vi "BSCAN_DEMO08_Zynq_W25Q128JV_registerRead_DeviceID_90h.vi"(8 "error in":errorcluster) -> (0 "error out":errorcluster, 4 "Data out":u8[](array[numeric]) format="%08b")   [LabVIEW 2017]
uses:
  Saldigi_protocol_library.lvlibp/SPI1_bitstream/SPI1_typedef.ctl
  Saldigi_protocol_library.lvlibp/HAL/HAL_version_typedef.ctl
  Saldigi_protocol_library.lvlibp
panel:
  in  "SPI1 typedef in":T1={"MOSI padded"=[], "CLK padded"=[], "-CS padded"=[], "String array"=[], "clocked bits"=0, "output rate"=0.0, "MOSI IO0 channel name"="chain0/xc7z020_clg400/PS_MIO2", "CLK channel name"="chain0/xc7z020_clg400/PS_MIO6", "MISO IO1 channel name"="chain0/xc7z020_clg400/PS_MIO3", "Parameter string"="", "-CS channel name"="chain0/xc7z020_clg400/PS_MIO1", "SPI mode"=enum."MODE 0", "Version"=enum."BSCAN V2"}
  in  "milliseconds to wait\nbetween iterations":u32
  out "dt":dbl(graph)=0.7297572000024957
  in  "stop":bool
  out "(ID7 - ID0) 17h":u8=23 format="%08b"
  out "(MF7 - MF0) EFh":u8=239 format="%08b"
  # "expected register values\nfrom datasheet"
  # "saldigi.fi protocol library"
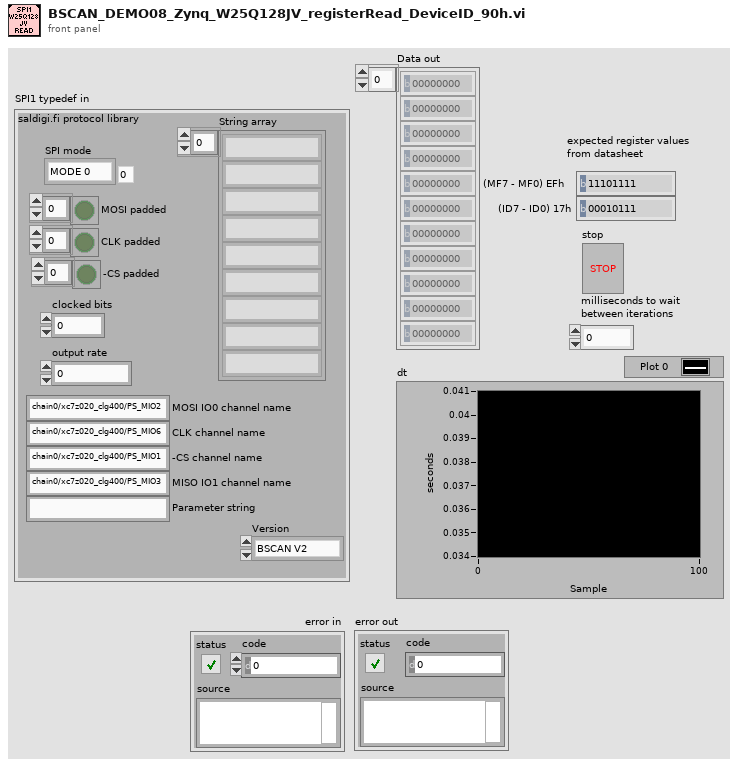
[diagram p1: front panel]
types:
  T1 = typedef "Saldigi_protocol_library.lvlibp/SPI1_typedef.ctl" = cluster{"MOSI padded":bool[], "CLK padded":bool[], "-CS padded":bool[], "String array":string[], "clocked bits":i32, "output rate":dbl, "MOSI IO0 channel name":string, "CLK channel name":string, "MISO IO1 channel name":string, "Parameter string":string, "-CS channel name":string, "SPI mode":enum16{"MODE 0", "MODE 1", "MODE 2", "MODE 3"}, "Version":T2}
  T2 = typedef "Saldigi_protocol_library.lvlibp/HAL_version_typedef.ctl" = enum16{"DAQmx V1", "DAQmx V2", "FTn232H", "BSCAN V1", "DAQmx V1.1", "DAQmx V2.1", "J-LINK BSCAN", "BSCAN V2"}
  T3 = enum16{"Write Enable 06h", "Volatile SR Write Enable 50h", "Write Disable 04h", "Release Power-down / ID ABh", "Manufacturer/Device ID 90h", "JEDEC ID 9Fh", "Read Unique ID 4Bh", "Read Data 03h", "Fast Read 0Bh", "Page Program 02h", "Sector Erase (4KB) 20h", "Block Erase (32KB) 52h", "Block Erase (64KB) D8h", "Chip Erase C7h/60h  ", "Read Status Register-1 05h", "Write Status Register-1 01h", "Read Status Register-2 35h", "Write Status Register-2 31h", "Read Status Register-3 15h", "Write Status Register-3 11h", "Read SFDP Register 5Ah", "Erase Security Register 44h", "Program Security Register 42h", "Read Security Register 48h", "Global Block Lock 7Eh", "Global Block Unlock 98h", "Read Block Lock 3Dh", "Individual Block Lock 36h", "Individual Block Unlock 39h", "Erase / Program Suspend 75h", "Erase / Program Resume 7Ah", "Power-down B9h", "Enable Reset 66h", "Reset Device 99h", "Fast Read Dual Output 3Bh", "Fast Read Dual I/O BBh", "Mftr./Device ID Dual I/O 92h", "Quad Input Page Program 32h", "Fast Read Quad Output 6Bh", "Mftr./Device ID Quad I/O 94h", "Fast Read Quad I/O Ebh", "Set Burst with Wrap 77h"}
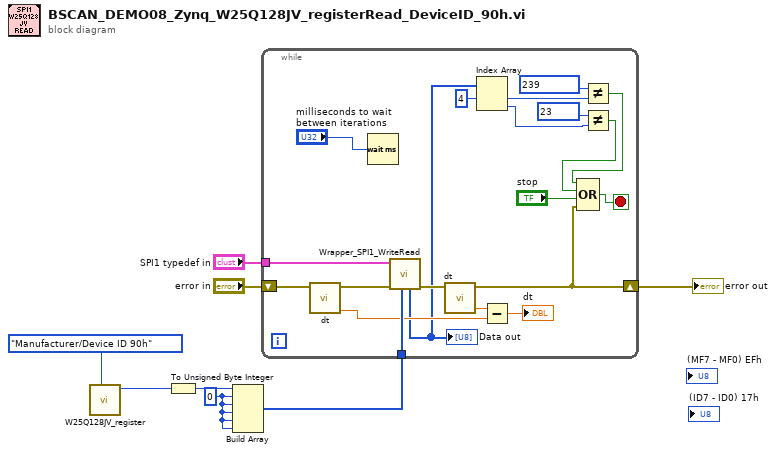
[diagram p0: block diagram]
diagram:
  w3 = u8 0 ("element")
  n1 = call "W25Q128JV_register.vi"("W25Q128JV register in"=T3."Manufacturer/Device ID 90h") -> ("W25Q128JV register address out"=w7:u32)  [unwired: 10 in]
  n2 = To Unsigned Byte Integer(number=w7) -> (unsigned 8bit integer=w8:u8)
  n3 = Build Array(w8, w3, w3, w3, w3, w3) -> (w4:u8[])
  n4 = while {
    tunnel: w4 -> [w28]
    shift-right: [w19] -> w5
    shift-left: "error in" -> [w27]
    tunnel: "SPI1 typedef in" -> [w9]
    stop <- w21 stop-if-true
    n5 = call "dt.vi"("error in"=w27) -> ("relative seconds"=w23:dbl, "error out"=w26:errorcluster)  [unwired: 9 in]
    n6 = Wait (ms)(milliseconds to wait="milliseconds to wait\nbetween iterations") -> ()  [unwired: 1 out]
    n7 = call "Wrapper_SPI1_WriteRead.vi"("Data in"=w28, "error in"=w26, "SPI1 typedef in"=w9) -> ("error out"=w25:errorcluster, "Data out"=w17:u8[])  [unwired: 6 in, 1 out]
    "Data out" <- w17
    n8 = call "dt.vi"("error in"=w25) -> ("relative seconds"=w24:dbl, "error out"=w19:errorcluster)  [unwired: 9 in]
    n9 = Index Array(array=w17, index #1=4 ("index")) -> (element #1=w15:u8, element #2=w12:u8)  [unwired: 1 in]
    n10 = Subtract(x=w24, y=w23) -> (x-y=→"dt":dbl)
    n11 = Not Equal?(x=u8 239, y=w15) -> (x != y?=w11:bool)
    n12 = Not Equal?(x=u8 23, y=w12) -> (x != y?=w10:bool)
    n13 = Compound Arithmetic op=OR(w11, w10, "stop", w19) -> (w21:bool)
  }
  "error out" <- w5
